vi "Action Start Heating.vi"(8 "error in (no error)":errorcluster, 10 "Setpoint":dbl=1e-05, 11 "heater_parent in":refnum<class "heater_parent.lvclass">) -> (0 "error out":errorcluster, 3 "heater_parent out":refnum<class "heater_parent.lvclass">)   [LabVIEW 2020, in "polar_bear_plus_drivers.lvlib" / "heater_parent.lvclass"]
doc: "\"Starts\" the temperature controller by setting the temperature setpoint to the previous recorded temperature setpoint last time the heater was stopped. This previous setpoint is not retained between sessions. Alternatively, a setpoint can be provided to this VI, which will change the temperature setpoint on the device to the new value.\n\nThere is not a programmatic way to start heating, as it is controlled by a switch on the side of the Polar Bear device. The best we can do is programmatically set the temperature setpoint to a safe value and resume the previous setpoint at a later time."
uses:
  <instrlib>/RxnRover/Driver Polar Bear Plus/heater_parent/heater_parent.lvclass
  <instrlib>/RxnRover/Driver Polar Bear Plus/heater_parent/heater_parent.lvclass/heater_parent.ctl
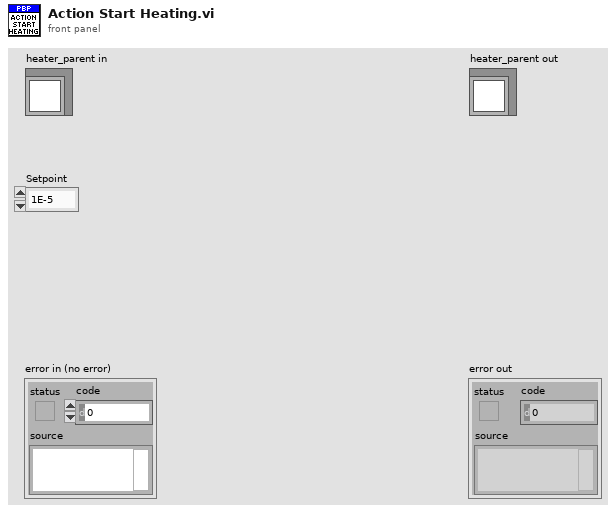
[diagram p1: front panel]
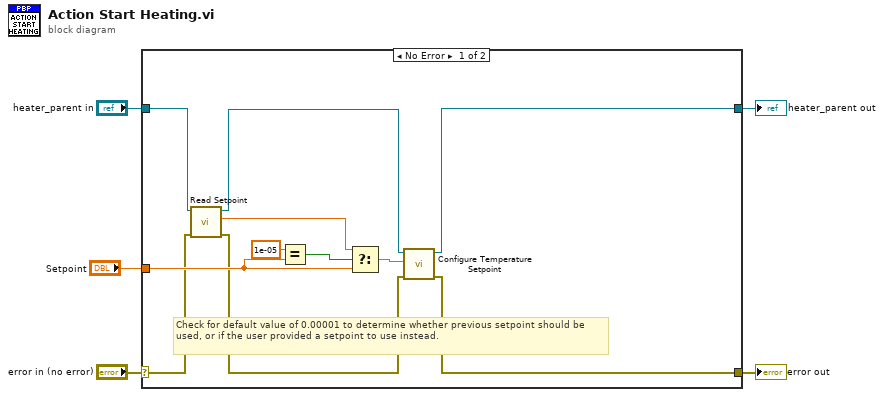
[diagram p0: block diagram]
diagram:
  n1 = case shown="No Error" "error in (no error)" {
    selector: "error in (no error)" -> [w9 w18]
    tunnel: [w16 w18] -> w4
    tunnel: [w15 w17] -> w2
    tunnel: "heater_parent in" -> [w11 w17]
    tunnel: "Setpoint" -> [w13 _]
    frame No Error {
      # "Check for default value of 0.00001 to determine whether previous setpoint should be used, or if the user provided a setpoint to use instead."
      n2 = call-dynamic "Read Setpoint.vi"("error in (no error)"=w9, "heater_parent in"=w11) -> ("error out"=w8:errorcluster, "Setpoint"=w7:dbl, "heater_parent out"=w10:refnum<class "heater_parent.lvclass">)  [unwired: 7 in]
      n3 = Equal?(x=1e-05, y=w13) -> (x = y?=w14:bool)
      n4 = Select(t=w7, s=w14, f=w13) -> (s? t:f=w12:dbl)
      n5 = call-dynamic "Configure Temperature Setpoint.vi"("error in (no error)"=w8, "New Setpoint"=w12, "heater_parent in"=w10) -> ("error out"=w16:errorcluster, "heater_parent out"=w15:refnum<class "heater_parent.lvclass">)  [unwired: 7 in]
    }
    frame Error {
    }
  }
  "error out" <- w4
  "heater_parent out" <- w2
